vi "TestLog.Record.vi"(7 "Mark":string, 8 "错误输入（无错误）":errorcluster, 10 "Info":string, 11 "TestLog_Recorder":refnum<queue>) -> (0 "错误输出":errorcluster, 3 "Input_ok?":bool)   [LabVIEW 2012, in "Lib_UEL.ATE.lvlib" / "Lib_Report.lvlib"]
uses:
  Lib_Report.lvlib
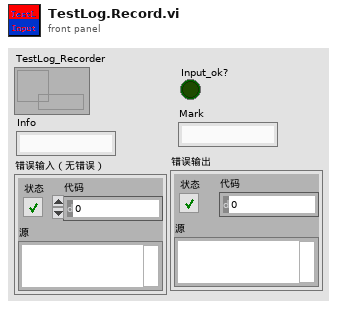
[diagram p1: front panel]
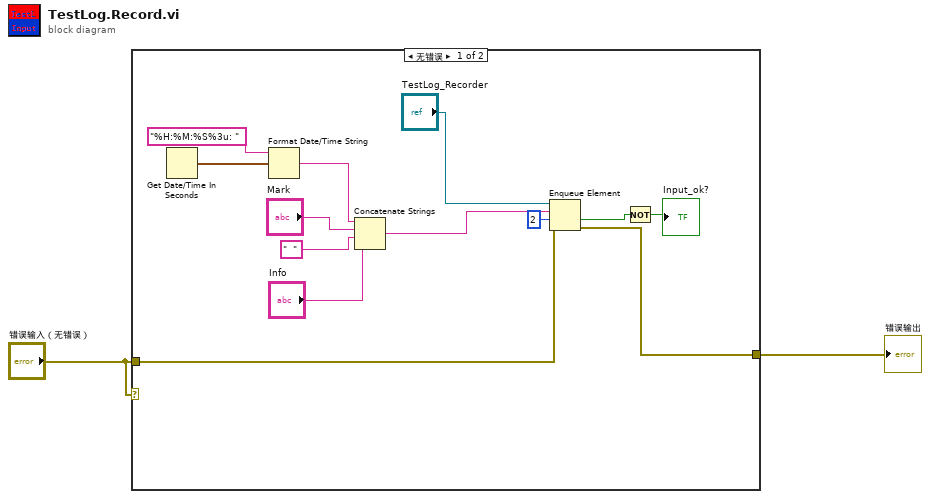
[diagram p0: block diagram]
diagram:
  n1 = case shown="无错误" "错误输入（无错误）" {
    selector: "错误输入（无错误）" -> [_ w16]
    tunnel: "错误输入（无错误）" -> [w6 _]
    tunnel: [w5 w16] -> w2
    frame No Error {
      n2 = Get Date/Time In Seconds() -> (seconds since 1Jan1904=w14:timestamp)
      n3 = Format Date/Time String(time format string (%c)="%H:%M:%S%3u: " ("时间格式字符串(%c)"), seconds (now)=w14) -> (date/time string=w12:string)  [unwired: 1 in]
      n4 = Concatenate Strings(w12, "Mark", "  " ("时间格式字符串(%c)"), "Info") -> (w8:string)
      n5 = Enqueue Element(queue="TestLog_Recorder", element=w8, timeout in ms (-1)=2 ("超时毫秒(-1)"), error in (no error)=w6) -> (timed out?=w3:bool, error out=w5:errorcluster)  [unwired: 1 out]
      n6 = Not(x=w3) -> (.not. x?=→"Input_ok?":bool)
    }
    frame Error {
    }
  }
  "错误输出" <- w2
